vi "MCS connecté.vi"(8 "error in (no error)":errorcluster caption="entrée d'erreur (pas d'erreur)", 11 "UI SA en entrée":refnum<class "UI SmarAct.lvclass">) -> (0 "error out":errorcluster caption="sortie d'erreur", 3 "UI SA en sortie":refnum<class "UI SmarAct.lvclass">)   [LabVIEW 2024, in "UI SmarAct.lvclass"]
uses:
  UI SmarAct.lvclass
  UI SmarAct.lvclass/UI SmarAct.ctl
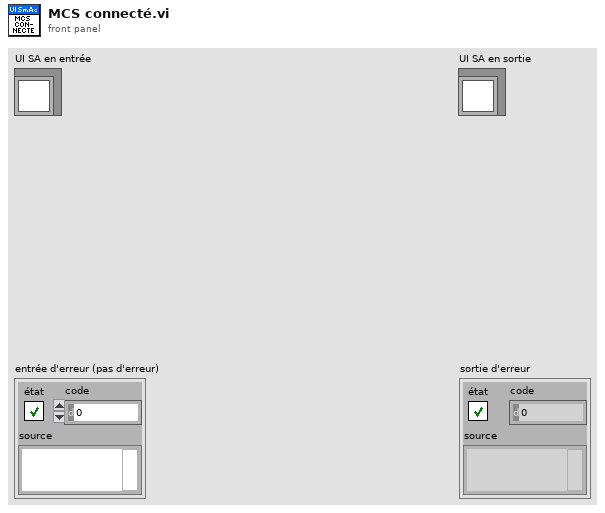
[diagram p1: front panel]
types:
  T1 = enum8{"Enabled", "Disabled", "Disabled and Grayed Out"}
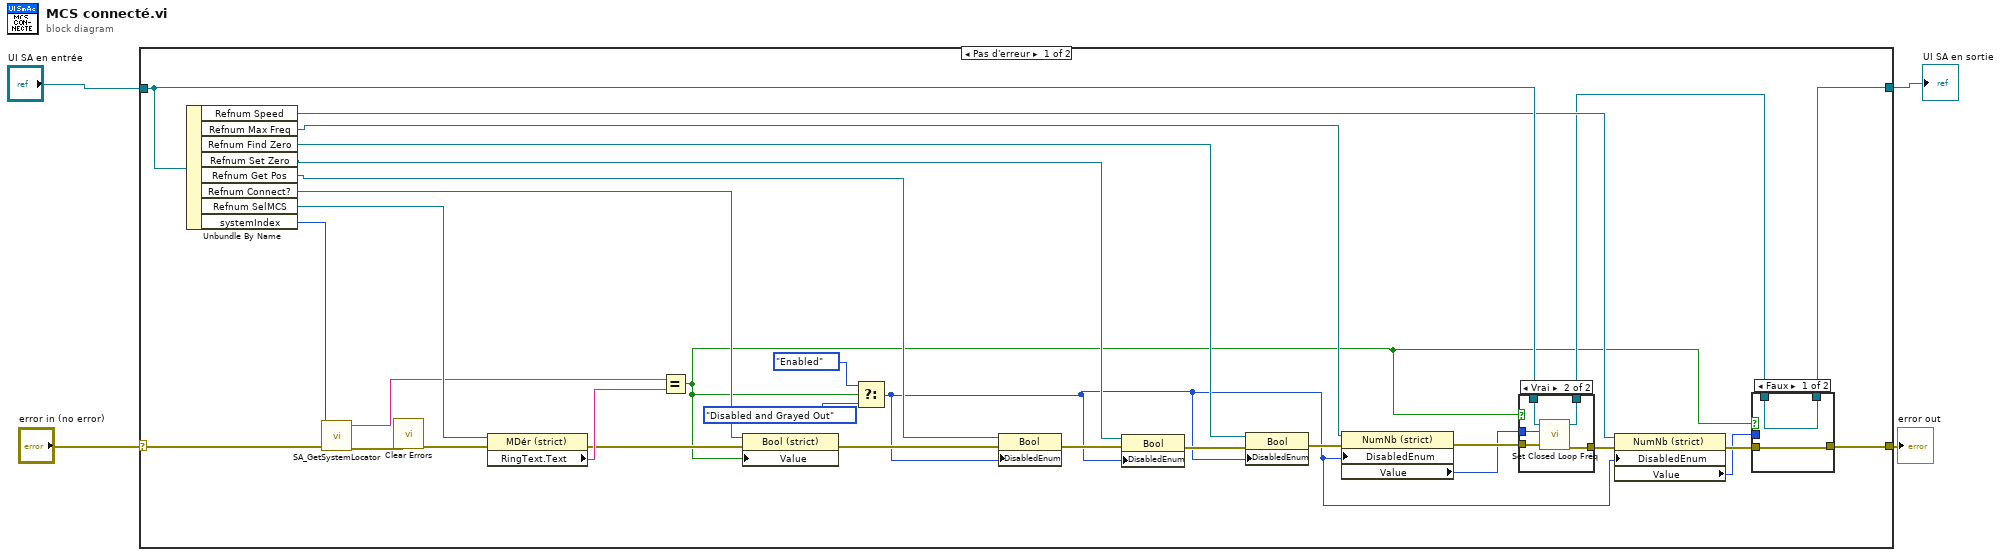
[diagram p0: block diagram]
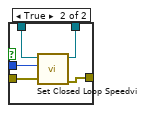
[diagram p2: hidden frame]
diagram:
  n1 = case shown="Pas d'erreur" "error in (no error)" {
    selector: "error in (no error)" -> [w35 w51]
    tunnel: [w10 w51] -> w3
    tunnel: [w7 w50] -> w1
    tunnel: "UI SA en entrée" -> [w15 w50]
    frame No Error {
      n2 = Unbundle By Name(w15) -> ("Refnum Speed"=w12:refnum<vi>, "Refnum Max Freq"=w18:refnum<vi>, "Refnum Find Zero"=w20:refnum<vi>, "Refnum Set Zero"=w22:refnum<vi>, "Refnum Get Pos"=w26:refnum<vi>, "Refnum Connect?"=w33:refnum<vi>, "Refnum SelMCS"=w32:refnum<vi>, "systemIndex"=w34:u32)
      n3 = call <vilib>:"SA_GetSystemLocator.vi"("systemIndex"=w34, "error in (no error)"=w35) -> ("error out"=w29:errorcluster, "systemLocator"=w31:string)  [unwired: 8 in]
      n4 = call <vilib>:"Clear Errors.vi"("error in (no error)"=w29) -> ("error out"=w28:errorcluster)  [unwired: 5 in, 1 out]
      n5 = property class="MDér (strict)"(reference=w32, error in=w28) -> (error out=w27:errorcluster, "RingText.Text"=w30:string)  [unwired: 1 out]
      n6 = Equal?(x=w31, y=w30) -> (x = y?=w6:bool)
      n7 = property class="Bool (strict)"(reference=w33, error in=w27, "Value"=w6) -> (error out=w23:errorcluster)  [unwired: 1 out]
      n8 = Select(t=T1."Enabled" ("Désactivée"), s=w6, f=T1."Disabled and Grayed Out" ("Désactivée")) -> (s? t:f=w5:T1)
      n9 = property class="Bool"(reference=w26, error in=w23, "DisabledEnum"=w5) -> (error out=w21:errorcluster)  [unwired: 1 out]
      n10 = property class="Bool"(reference=w22, error in=w21, "DisabledEnum"=w5) -> (error out=w19:errorcluster)  [unwired: 1 out]
      n11 = property class="Bool"(reference=w20, error in=w19, "DisabledEnum"=w5) -> (error out=w17:errorcluster)  [unwired: 1 out]
      n12 = property class="NumNb (strict)"(reference=w18, error in=w17, "DisabledEnum"=w5) -> (error out=w16:errorcluster, "Value"=w14:u32)  [unwired: 1 out]
      n13 = case shown="Vrai" w6 {
        tunnel: w16 -> [w44 w49]
        tunnel: [w44 w48] -> w13
        tunnel: w15 -> [w43 w47]
        tunnel: [w43 w46] -> w8
        tunnel: w14 -> [_ w45]
        frame False {
        }
        frame True {
          n14 = call "Set Closed Loop Fréq.vi"("error in (no error)"=w49, "frequency"=w45, "UI SA en entrée"=w47) -> ("error out"=w48:errorcluster, "UI SA en sortie"=w46:refnum<class "UI SmarAct.lvclass">)  [unwired: 7 in]
        }
      }
      n15 = property class="NumNb (strict)"(reference=w12, error in=w13, "DisabledEnum"=w5) -> (error out=w11:errorcluster, "Value"=w9:u32)  [unwired: 1 out]
      n16 = case shown="Faux" w6 {
        tunnel: w11 -> [w36 w42]
        tunnel: [w36 w41] -> w10
        tunnel: w9 -> [_ w40]
        tunnel: w8 -> [w37 w39]
        tunnel: [w37 w38] -> w7
        frame False {
        }
        frame True {
          n17 = call "Set Closed Loop Speedvi.vi"("error in (no error)"=w42, "speed"=w40, "UI SA en entrée"=w39) -> ("error out"=w41:errorcluster, "UI SA en sortie"=w38:refnum<class "UI SmarAct.lvclass">)  [unwired: 7 in]
        }
      }
    }
    frame Error {
    }
  }
  "error out" <- w3
  "UI SA en sortie" <- w1
